vi "Build Graph.vi"(8 "error in (no error)":errorcluster, 11 "CalibReport in":refnum<class "CalibReport.lvclass">) -> (0 "error out":errorcluster, 2 "CalibPoints":cluster{dbl[], dbl[]}(graph), 3 "CalibReport out":refnum<class "CalibReport.lvclass">)   [LabVIEW 2024, in "CalibReport.lvclass"]
uses:
  CalibReport.lvclass
  CalibReport.lvclass/CalibReport.ctl
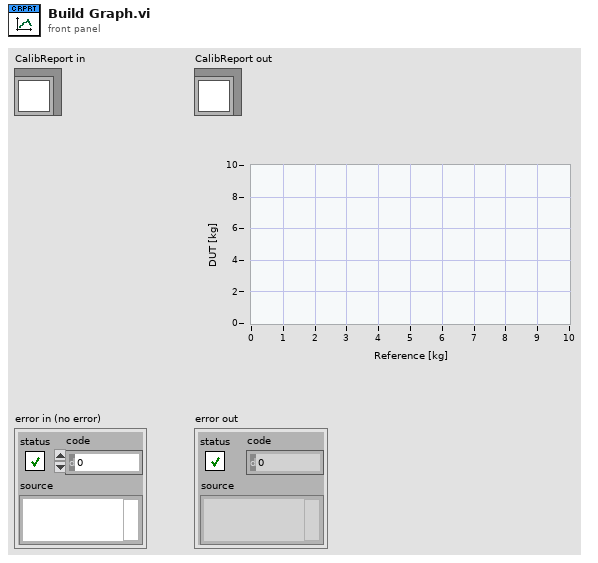
[diagram p1: front panel]
types:
  T1 = typedef "cReportEntry.ctl" = cluster{"Reference [kg]":dbl, "DUT value [kg]":dbl}
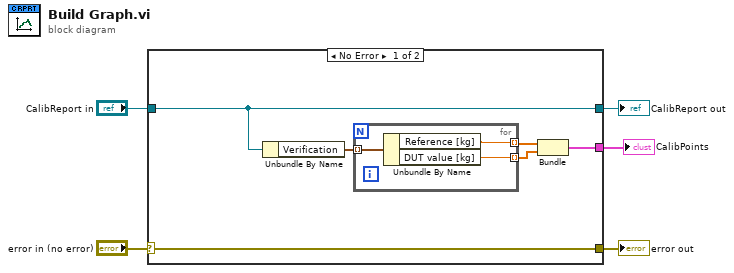
[diagram p0: block diagram]
diagram:
  n1 = case shown="No Error" "error in (no error)" {
    selector: "error in (no error)" -> [w11 w16]
    tunnel: [w11 w16] -> w4
    tunnel: [w10 w15] -> w2
    tunnel: "CalibReport in" -> [w10 w15]
    tunnel: [w6 _] -> w1
    frame No Error {
      n2 = Unbundle By Name(w10) -> ("Verification"=w9:T1[])
      n3 = for {
        tunnel: w9 -> [w14] mode=indexing
        tunnel: [w13] -> w8 mode=indexing
        tunnel: [w12] -> w7 mode=indexing
        n4 = Unbundle By Name(w14) -> ("Reference [kg]"=w13:dbl, "DUT value [kg]"=w12:dbl)
      }
      n5 = Bundle(w8, w7) -> (w6:cluster{dbl[], dbl[]})  [unwired: 1 in]
    }
    frame Error {
    }
  }
  "error out" <- w4
  "CalibReport out" <- w2
  "CalibPoints" <- w1
